vi "MGI Write Key (Double[]).vi"(7 "Section":string, 8 "error in (no error)":errorcluster, 9 "Value[]":dbl[](array[numeric]) format="%.2f", 10 "Key":string, 11 "Refnum":T1) -> (0 "error out":errorcluster, 3 "Refnum":T1)   [LabVIEW 2016]
doc: "Write a 1D float array in a human readable format. The \"key\" is actually placed in a separate section.\n\n\nAuthored by David A. Moore\nsupport@mooregoodideas.com\nwww.mooregoodideas.com\n\nCopyright (c) 2010, Moore Good Ideas, Inc.\n\nAll rights reserved.\n\nRedistribution and use in source and binary forms, with or without modification, are permitted provided that the following conditions are met:\n\n * Redistributions of source code must retain the above copyright notice, this list of conditions and the following disclaimer.\n * Redistributions in binary form must reproduce the above copyright notice, this list of conditions and the following disclaimer in the documentation and/or other materials provided with the distribution.\n * Neither the name of Moore Good Ideas, Inc. nor the names of its contributors may be used to endorse or promote products derived from this software without specific prior written permission.\n\nTHIS SOFTWARE IS PROVIDED BY THE COPYRIGHT HOLDERS AND CONTRIBUTORS \"AS IS\" AND ANY EXPRESS OR IMPLIED WARRANTIES, INCLUDING, BUT NOT LIMITED TO, THE IMPLIED WARRANTIES OF MERCHANTABILITY AND FITNESS FOR A PARTICULAR PURPOSE ARE DISCLAIMED. IN NO EVENT SHALL THE COPYRIGHT OWNER OR CONTRIBUTORS BE LIABLE FOR ANY DIRECT, INDIRECT, INCIDENTAL, SPECIAL, EXEMPLARY, OR CONSEQUENTIAL DAMAGES (INCLUDING, BUT NOT LIMITED TO, PROCUREMENT OF SUBSTITUTE GOODS OR SERVICES; LOSS OF USE, DATA, OR PROFITS; OR BUSINESS INTERRUPTION) HOWEVER CAUSED AND ON ANY THEORY OF LIABILITY, WHETHER IN CONTRACT, STRICT LIABILITY, OR TORT (INCLUDING NEGLIGENCE OR OTHERWISE) ARISING IN ANY WAY OUT OF THE USE OF THIS SOFTWARE, EVEN IF ADVISED OF THE POSSIBILITY OF SUCH DAMAGE."
uses:
  <vilib>/Utility/config.llb/Config Data RefNum.ctl
  <vilib>/Utility/config.llb/Write Key (I32).vi
  <vilib>/Utility/config.llb/Write Key (Double).vi
  <vilib>/Utility/config.llb/NI_LVConfig.lvlib
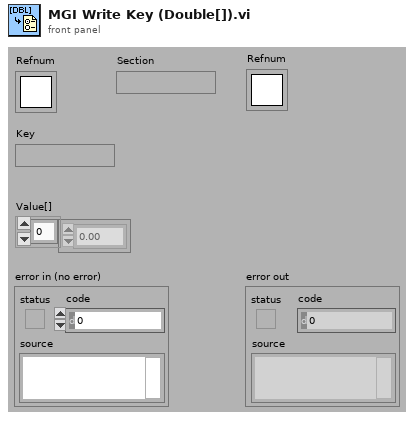
[diagram p1: front panel]
types:
  T1 = typedef "NI_LVConfig.lvlib/Config Data RefNum.ctl" = refnum<k1>
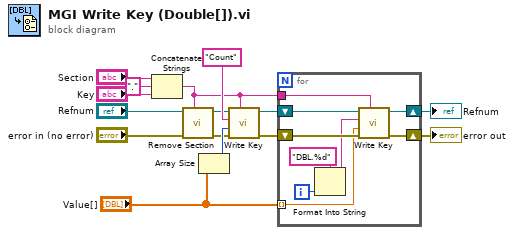
[diagram p0: block diagram]
diagram:
  n1 = Concatenate Strings("Section", "." ("Substring"), "Key") -> (w2:string)
  n2 = call <vilib>:"Remove Section.vi"("section"=w2, "error in (no error)"="error in (no error)", "refnum"="Refnum") -> ("error out"=w5:errorcluster, "refnum out"=w1:T1)  [unwired: 6 in, 1 out]
  n3 = Array Size(array="Value[]") -> (size(s)=w15:i32)
  n4 = call-poly <vilib>:"Write Key.vi"("section"=w2, "error in (no error)"=w5, "value"=w15, "key"="Count", "refnum"=w1) -> ("error out"=w12:errorcluster, "refnum out"=w11:T1)  [unwired: 4 in, 1 out]
  n5 = for {
    tunnel: "Value[]" -> [w22] mode=indexing
    shift-right: [w20] -> w10
    shift-left: w12 -> [w24]
    shift-right: [w19] -> w9
    shift-left: w11 -> [w23]
    tunnel: w2 -> [w21]
    i -> [w18]
    n6 = Format Into String(format string="DBL.%d" ("Format String"), w18) -> (resulting string=w17:string)  [unwired: 2 in, 1 out]
    n7 = call-poly <vilib>:"Write Key.vi"("section"=w21, "error in (no error)"=w24, "value"=w22, "key"=w17, "refnum"=w23) -> ("error out"=w20:errorcluster, "refnum out"=w19:T1)  [unwired: 4 in, 1 out]
  }
  "error out" <- w10
  "Refnum" <- w9
